vi "Exercise 6.4.vi"() -> ()   [LabVIEW 2020]
panel:
  out "Captured Spectrum Out":dbl[](array[numeric])
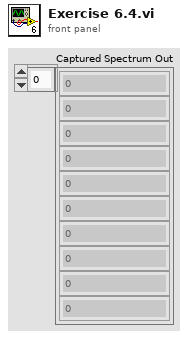
[diagram p1: front panel]
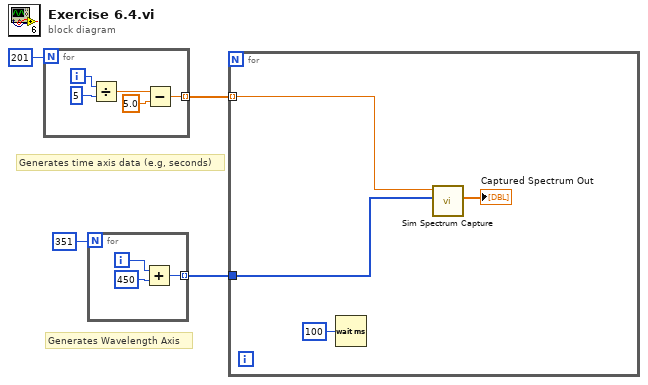
[diagram p0: block diagram]
diagram:
  # "Generates time axis data (e.g, seconds)"
  # "Generates Wavelength Axis"
  n1 = for {
    N: 201 -> [_]
    tunnel: [w5] -> w1 mode=indexing
    i -> [w9]
    n2 = Divide(x=w9, y=5) -> (x/y=w7:dbl)
    n3 = Subtract(x=w7, y=5.0) -> (x-y=w5:dbl)
  }
  n4 = for {
    N: 351 -> [_]
    tunnel: [w10] -> w3 mode=indexing
    i -> [w12]
    n5 = Add(x=w12, y=450) -> (x+y=w10:i32)
  }
  n6 = for {
    tunnel: w3 -> [w14]
    tunnel: w1 -> [w16] mode=indexing
    n7 = Wait (ms)(milliseconds to wait=u32 100) -> ()  [unwired: 1 out]
    n8 = call "Sim Spectrum Capture.vi"("Wavelength Axis"=w14, "Time Point"=w16) -> ("Captured Spectrum Out"=→"Captured Spectrum Out":dbl[])  [unwired: 9 in]
  }
